vi "FTS GetSet Acquisition Option Spectrum Smoothing.vi"(0 "spectrIdx":u16, 5 "channel":u16, 7 "smoothingType":u16, 9 "width":u16, 11 "nrOfPasses":u16, 12 "readWrite":enum16{"read", "write"}(ring)) -> (4 "FTSLib status":i32, 8 "smoothingType":u16, 10 "width read":u16, 15 "nrOfPAsses read":u16)   [LabVIEW 2010, in "FTSLib.lvlib"]
uses:
  FTSLib.lvlib
  FTSLib.dll
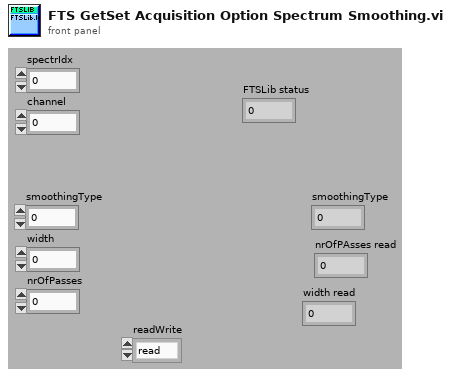
[diagram p1: front panel]
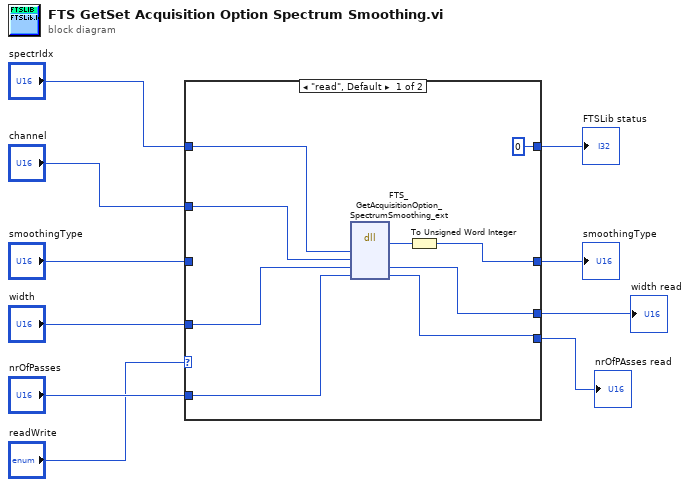
[diagram p0: block diagram]
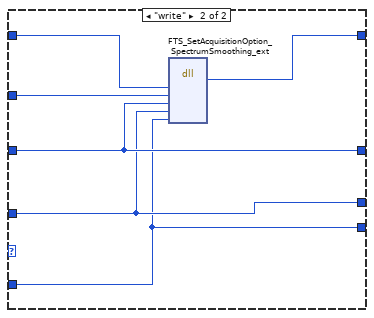
[diagram p2: hidden frame]
diagram:
  n1 = case shown="\"read\", Default" "readWrite" {
    tunnel: "channel" -> [w18 w24]
    tunnel: "spectrIdx" -> [w19 w25]
    tunnel: "smoothingType" -> [_ w22]
    tunnel: "width" -> [w17 w21]
    tunnel: "nrOfPasses" -> [w15 w20]
    tunnel: [0 ("return type") w23] -> w4
    tunnel: [w11 w22] -> w3
    tunnel: [w14 w21] -> w2
    tunnel: [w13 w20] -> w1
    frame "read", Default {
      n2 = dll-call lib="FTSLib.dll" fn="FTS_GetAcquisitionOption_SpectrumSmoothing_ext"("spectrIdx"=w19, "channel"=w18, "width"=w17, "nrOfPAsses"=w15) -> ("return type"=w12:i32, "width"=w14:u16, "nrOfPAsses"=w13:u16)  [unwired: 5 in, 2 out]
      n3 = To Unsigned Word Integer(number=w12) -> (unsigned 16bit integer=w11:u16)
    }
    frame "write" {
      n4 = dll-call lib="FTSLib.dll" fn="FTS_SetAcquisitionOption_SpectrumSmoothing_ext"("spectrIdx"=w25, "channel"=w24, "smoothingType"=w22, "width"=w21, "nrOfPasses"=w20) -> ("return type"=w23:i32)  [unwired: 8 in, 2 out]
    }
  }
  "FTSLib status" <- w4
  "smoothingType" <- w3
  "width read" <- w2
  "nrOfPAsses read" <- w1
